vi "SlideTiles.vi"(7 "Side":T1=enum."left", 8 "error in (no error)":errorcluster, 10 "Tilecodes":u32[](array[numeric])) -> (0 "error out":errorcluster)   [LabVIEW 2019, in "RT_Game.lvlib" / "Engine.lvclass"]
uses:
  Engine.lvclass
  ScreenSide.ctl
  MessageCluster.ctl
  SlideJob.ctl
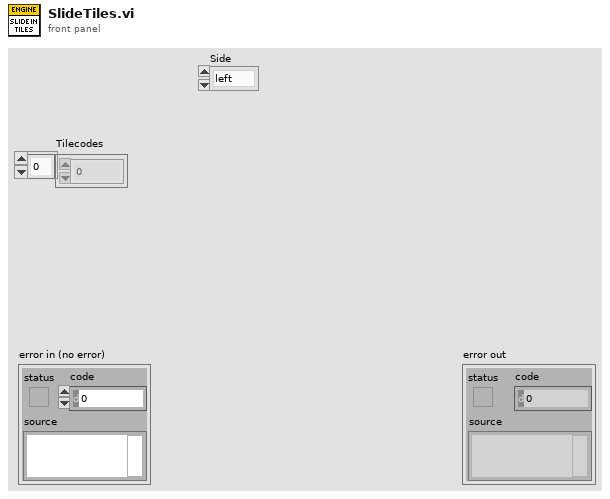
[diagram p1: front panel]
types:
  T1 = typedef "RT_Game.lvlib/Engine.lvclass/ScreenSide.ctl" = enum16{"up", "down", "left", "right", "none"}
  T2 = typedef "RT_Game.lvlib/Engine.lvclass/SlideJob.ctl" = cluster{"Pixel":u32[], "Side":T1}
  T3 = typedef "RT_Game.lvlib/Engine.lvclass/MessageCluster.ctl" = cluster{"Message":string, "Data":variant}
  T4 = typedef "RT_Game.lvlib/Engine.lvclass/Queues.ctl" = cluster{"MusicQueue":refnum<queue>, "TilesQueue":refnum<queue>, "SoundsQueue":refnum<queue>}
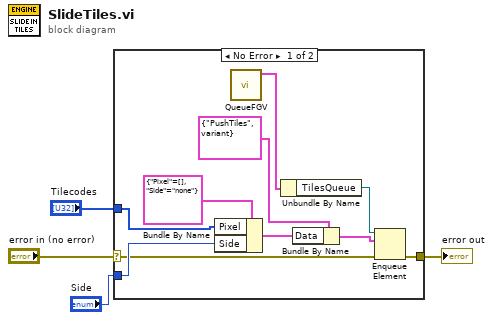
[diagram p0: block diagram]
diagram:
  n1 = case shown="No Error" "error in (no error)" {
    selector: "error in (no error)" -> [w12 w15]
    tunnel: [w11 w15] -> w3
    tunnel: "Side" -> [w14 _]
    tunnel: "Tilecodes" -> [w13 _]
    frame No Error {
      n2 = Bundle By Name(cluster=T2 {"Pixel"=[], "Side"=enum."none"} ("SlideJob"), "Pixel"=w13, "Side"=w14) -> (w7:T2)
      n3 = call "QueueFGV.vi"() -> ("Queues out"=w6:T4)  [unwired: 10 in, 1 out]
      n4 = Unbundle By Name(w6) -> ("TilesQueue"=w5:refnum<queue>)
      n5 = Bundle By Name(cluster=T3 {"Message"="PushTiles", "Data"=variant} ("element"), "Data"=w7) -> (w9:T3)
      n6 = Enqueue Element(queue=w5, element=w9, error in (no error)=w12) -> (error out=w11:errorcluster)  [unwired: 1 in, 2 out]
    }
    frame Error {
    }
  }
  "error out" <- w3
